vi "Bool til status.vi"(1 "Force NA(F)":bool, 2 "Boolean":bool) -> (7 "Status":T1)   [LabVIEW 2011]
uses:
  Status Digitalish.ctl
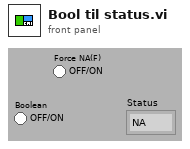
[diagram p1: front panel]
types:
  T1 = typedef "Status Digitalish.ctl" = enum16{"NA", "False", "True"}
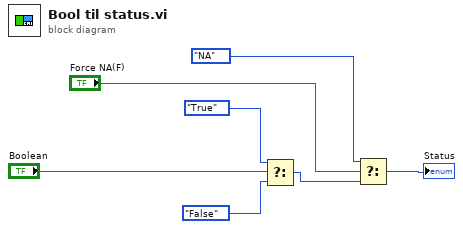
[diagram p0: block diagram]
diagram:
  n1 = Select(t=Status_Digitalish."True" ("Value"), s="Boolean", f=Status_Digitalish."False" ("Value")) -> (s? t:f=w4:T1)
  n2 = Select(t=Status_Digitalish."NA" ("Value"), s="Force NA(F)", f=w4) -> (s? t:f=→"Status":T1)
